vi "Packet Governor.vi"(0 "ready for input? in":T1, 5 "start packet":bool, 7 "minimum packet interval":u32=1) -> (4 "ready for input? out":T1)   [LabVIEW 2017, in "My Network FPGA v1.lvlib"]
uses:
  My Network FPGA v1.lvlib
  <instrlib>/_niInstr/Basic Elements/v1/FPGA/Private/Count Down U32.vi
  <instrlib>/_niInstr/Basic Elements/v1/FPGA/niInstr Basic Elements v1 FPGA.lvlib
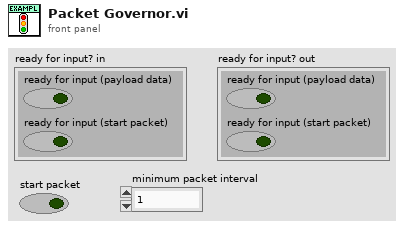
[diagram p1: front panel]
types:
  T1 = cluster{"ready for input (payload data)":bool, "ready for input (start packet)":bool}
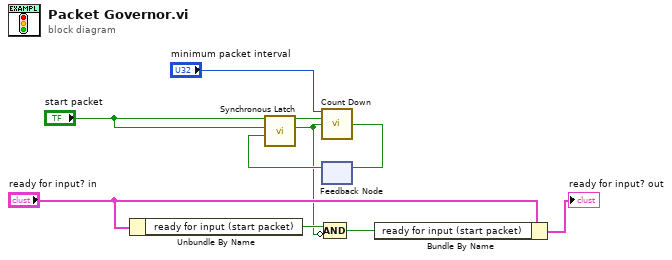
[diagram p0: block diagram]
diagram:
  n1 = Unbundle By Name("ready for input? in") -> ("ready for input (start packet)"=w3:bool)
  n2 = feedback #1() -> (w7:bool)  [unwired: 1 in]
  n3 = call <instrlib>:"Synchronous Latch.vi"("clear"=w7, "set"="start packet") -> ("out"=w2:bool)  [unwired: 9 in]
  n4 = call-poly <instrlib>:"Count Down.vi"("count in"="minimum packet interval", "load"="start packet", "decrement"=w2) -> ("terminal count"=w8:bool)  [unwired: 11 in, 1 out]
  n5 = feedback-in #1(w8) -> ()
  n6 = Compound Arithmetic op=AND(w3, invert w2) -> (w1:bool)
  n7 = Bundle By Name(cluster="ready for input? in", "ready for input (start packet)"=w1) -> (→"ready for input? out":T1)
